vi "Apply Reverse Proxy.vi"(8 "error in (no error)":errorcluster, 11 "OAuthAccessToken in":refnum<class "OAuthAccessToken.lvclass">) -> (0 "error out":errorcluster, 3 "OAuthAccessToken out":refnum<class "OAuthAccessToken.lvclass">)   [LabVIEW 2020, in "OAuthAccessToken.lvclass"]
uses:
  OAuthAccessToken.lvclass
  OAuth2 Token Element -- enum.ctl
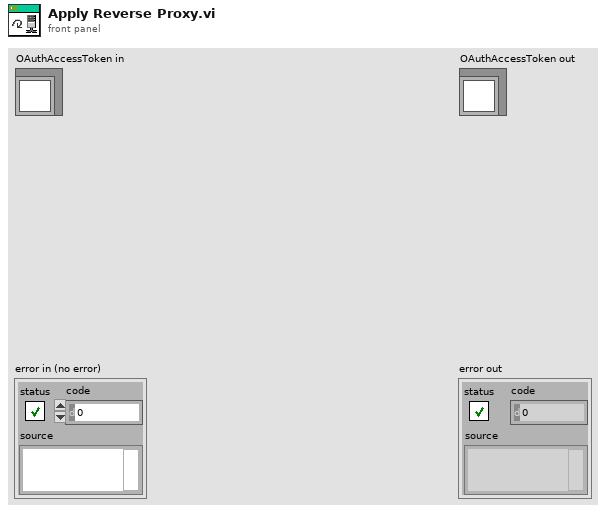
[diagram p1: front panel]
types:
  T1 = typedef "OAuthAccessToken.lvclass/OAuth2 Token Element -- enum.ctl" = enum16{"client_id", "client_secret", "response_type", "scope", "redirect_uri", "error", "error_description", "error_uri", "grant_type", "code", "access_token", "token_type", "expires_in", "username", "password", "refresh_token", "code_challenge", "code_challenge_method", "reverse_proxy_uri", "endpoint element"}
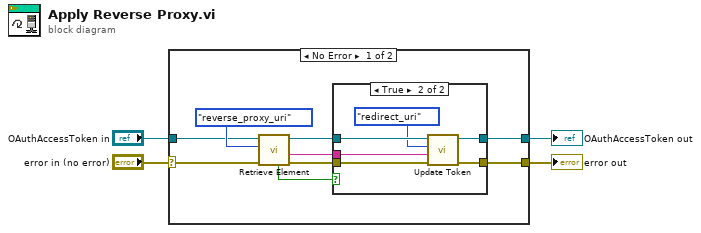
[diagram p0: block diagram]
diagram:
  n1 = case shown="No Error" "error in (no error)" {
    selector: "error in (no error)" -> [w6 w23]
    tunnel: [w5 w23] -> w3
    tunnel: [w8 w22] -> w1
    tunnel: "OAuthAccessToken in" -> [w9 w22]
    frame No Error {
      n2 = call "Retrieve Element.vi"("error in (no error)"=w6, "Token element"=OAuth2_Token_Element_--_enum."reverse_proxy_uri", "OAuthAccessToken in"=w9) -> ("error out"=w7:errorcluster, "Value"=w10:string, "OAuthAccessToken out"=w12:refnum<class "OAuthAccessToken.lvclass">, "element found"=w11:bool)  [unwired: 4 in, 1 out]
      n3 = case shown="True" w11 {
        tunnel: w12 -> [w15 w21]
        tunnel: [w15 w19] -> w8
        tunnel: w10 -> [_ w18]
        tunnel: w7 -> [w14 w17]
        tunnel: [w14 w16] -> w5
        frame False {
        }
        frame True {
          n4 = call "Update Token.vi"("error in (no error)"=w17, "Value"=w18, "Token element"=OAuth2_Token_Element_--_enum."redirect_uri", "OAuthAccessToken in"=w21) -> ("error out"=w16:errorcluster, "OAuthAccessToken out"=w19:refnum<class "OAuthAccessToken.lvclass">)  [unwired: 6 in]
        }
      }
    }
    frame Error {
    }
  }
  "error out" <- w3
  "OAuthAccessToken out" <- w1
